vi "DiffDriveDashWrite.vi"   [LabVIEW 2025]
uses:
  DiffDriveGlobals.vi
  <vilib>/Rock Robotics/Network Tables/NT Write Number.vi
  <vilib>/Rock Robotics/Network Tables/NT Write Boolean.vi
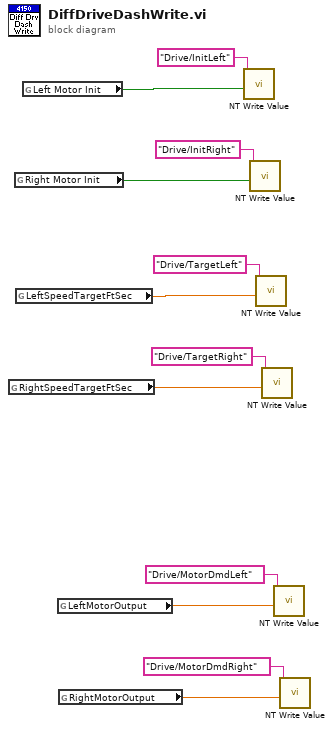
[diagram p0: block diagram]
diagram:
  n1 = global read "DiffDriveGlobals.vi" "RightSpeedTargetFtSec"() -> (w9:dbl)
  n2 = global read "DiffDriveGlobals.vi" "Right Motor Init"() -> (w1:bool)
  n3 = global read "DiffDriveGlobals.vi" "LeftSpeedTargetFtSec"() -> (w10:dbl)
  n4 = global read "DiffDriveGlobals.vi" "Left Motor Init"() -> (w2:bool)
  n5 = global read "DiffDriveGlobals.vi" "LeftMotorOutput"() -> (w6:dbl)
  n6 = global read "DiffDriveGlobals.vi" "RightMotorOutput"() -> (w5:dbl)
  n7 = call-poly <vilib>:"NT Write Value.vi"("value"=w2, "name"="Drive/InitLeft") -> ()  [unwired: 9 in, 1 out]
  n8 = call-poly <vilib>:"NT Write Value.vi"("value"=w1, "name"="Drive/InitRight") -> ()  [unwired: 9 in, 1 out]
  n9 = call-poly <vilib>:"NT Write Value.vi"("value"=w10, "name"="Drive/TargetLeft") -> ()  [unwired: 9 in, 1 out]
  n10 = call-poly <vilib>:"NT Write Value.vi"("value"=w9, "name"="Drive/TargetRight") -> ()  [unwired: 9 in, 1 out]
  n11 = call-poly <vilib>:"NT Write Value.vi"("value"=w6, "name"="Drive/MotorDmdLeft") -> ()  [unwired: 9 in, 1 out]
  n12 = call-poly <vilib>:"NT Write Value.vi"("value"=w5, "name"="Drive/MotorDmdRight") -> ()  [unwired: 9 in, 1 out]
